vi "Perform Measurement.vi"(7 "MeasurementConfiguration":T2={"BandStart"=20.0, "BandStop"=20000.0, "Amplitude"=1.0, "Frequency"=1000.0, "FullScaleRange"=2.825, "DataLine"=0, "SampleRate"=12288000, "MeasurementDuration"=19200.0, "Channel"=0, "FrameSyncEdgeForChannel_0"=0, "ChannelCountPerFrame"=2, "ChannelLength"=32, "BitDepth"=24, "Channel_0_offset"=1, "Endianness"=0, "DataJustification"=0, "FrameSyncPulseWidth"=32, "BitClockEdgeSync"=1, "ClockRate"=0, "FrameLength"=0, "NumberOfWords"=0, "Sensitivity"=0.0}, 8 "Y":dbl[](array[numeric]), 9 "dt":dbl, 11 "WeightingFilter":string) -> (1 "error out":errorcluster, 2 "TimeDomain":dbl[](array[numeric]), 3 "Spectrum":dbl[](array[numeric]), 5 "MeasurementResults":T1)   [LabVIEW 2021]
uses:
  Measurement Configuration.ctl
  MeasurementResults.ctl
  <vilib>/addons/_NISVFA/_Shared subVIs/Controls/svc_Window.ctl
  <vilib>/addons/_NISVFA/_Shared subVIs/Common/SVL Set dB Reference (N Ch - 1 Ref).vi
  <vilib>/addons/Sound and Vibration/svt_Level/SVL AC & DC Level (Time) (N Ch).vi
  <vilib>/addons/Sound and Vibration/svt_Single Tone Measurements/SVT Spurious Free Dynamic Range (Frequency) (1 Ch).vi
  <vilib>/addons/_NISVFA/_Spectrum Processing/SVFA Unit Conversion (Complex) (1 Ch).vi
  <vilib>/addons/_NISVFA/_Shared subVIs/Common/SVL Set dB Reference (1 Ch).vi
  <vilib>/addons/Sound and Vibration/svt_Level/SVL AC & DC Level (Time) (1 Ch).vi
  <vilib>/addons/_NISVFA/_Spectrum Processing/SVFA Get Spectrum Subset.vi
  <vilib>/addons/_NISVFA/_Spectrum Processing/SVFA Get Spectrum Subset (Complex) (1 Ch).vi
  <vilib>/addons/_NISVFA/_Shared subVIs/Common/svc_Window Parameters.vi
  <vilib>/addons/_NISVFA/_Shared subVIs/Common/svc_Extract Single Tone Information (complex).vi
  <vilib>/addons/_NISVFA/_Shared subVIs/Common/svc_Check Frequency Range in Spectrum.vi
  <vilib>/addons/_NISVFA/_Spectrum Processing/SVFA Spectrum Peak Search.vi
  <vilib>/addons/_NISVFA/_Spectrum Processing/SVFA Spectrum Peak Search (1 Ch).vi
  <vilib>/addons/_NISVFA/_Shared subVIs/Common/svc_Spectrum Units.vi
  <vilib>/addons/_NISVFA/_Shared subVIs/Common/svc_Log View for Spectrum (1Ch).vi
  <vilib>/addons/_NISVFA/_Spectrum Processing/SVFA Unit Conversion (1 Ch).vi
  <vilib>/addons/_NISVFA/_Shared subVIs/Common/svc_Complex Datatype Defaults.vi
  <vilib>/addons/_NISVFA/_Shared subVIs/Common/svc_Build Unit Label for Frequency Range.vi
  <vilib>/addons/_NISVFA/_Shared subVIs/Common/SVL Set dB Reference (variant).vi
  <vilib>/addons/_NISVFA/_Shared subVIs/Common/svc_Get SV Channel Info.vi
  <vilib>/Analysis/baseanly.llb/Mean.vi
  <vilib>/Analysis/baseanly.llb/Mean (DBL).vi
  <vilib>/addons/_NISVFA/_Shared subVIs/Windowing/svfa_Scaled Time Domain Window (Array).vi
  <vilib>/addons/_NISVFA/_Spectrum Processing/SVFA Get Tone Amplitude and Phase (1 Ch).vi
  <vilib>/addons/_NISVFA/_Spectrum Processing/subVIs/svfa_Compute Complex Spectrum for Export.vi
  <vilib>/addons/_NISVFA/_Shared subVIs/Common/svc_Check Frequency Range in Bandwidth.vi
  <vilib>/addons/_NISVFA/_Shared subVIs/Common/svc_Convert Start and Stop to Start Index and Length.vi
  <vilib>/addons/_NISVFA/_Spectrum Processing/subVIs/svfa_Spectrum Peak Search.vi
  <vilib>/addons/_NISVFA/_Shared subVIs/Common/svc_Format Value (DBL).vi
  <vilib>/addons/_NISVFA/_Shared subVIs/Common/svc_Get Weighting Enum and Labels.vi
  <vilib>/addons/_NISVFA/_Shared subVIs/Common/svc_Engineering Units to Unit Label.vi
  <vilib>/addons/_NISVFA/_Shared subVIs/Common/svc_Surround NonAlpha String with Parentheses.vi
  <vilib>/dlg_ctls.llb/Space Constant.vi
  <vilib>/addons/_NISVFA/_Shared subVIs/Common/svc_Unwrap Phase.vi
  <vilib>/addons/_NISVFA/_Shared subVIs/Common/svc_Convert Spectrum Array to dB.vi
  <vilib>/addons/_NISVFA/_Spectrum Processing/subVIs/svfa_Conversion Utility (spectrum info).vi
  <vilib>/addons/_NISVFA/_Shared subVIs/Common/svc_Unit Label to Engineering Units.vi
  <vilib>/addons/_NISVFA/_Spectrum Processing/subVIs/svfa_Spectrum Info Window to windowTd Type Def.vi
  <vilib>/Analysis/4window.llb/Force Window.vi
  <vilib>/Analysis/4window.llb/Force Window (DBL).vi
  <vilib>/Analysis/4window.llb/Exponential Window.vi
  <vilib>/Analysis/4window.llb/Exponential Window (DBL).vi
  <vilib>/addons/_NISVFA/_Spectrum Processing/subVIs/svfa_Window Frequency Response.vi
  <vilib>/addons/_NISVFA/_Spectrum Processing/subVIs/svfa_Window Frequency Response (double array).vi
  <vilib>/Analysis/baseanly.llb/Dot Product.vi
  <vilib>/Analysis/baseanly.llb/Complex Dot Product.vi
  <vilib>/addons/_NISVFA/_Spectrum Processing/subVIs/svfa_Peak Rough Search Indices.vi
  <vilib>/addons/_NISVFA/_Shared subVIs/Common/svc_Unit Label Lexical Class.vi
  <vilib>/addons/_NISVFA/_Spectrum Processing/subVIs/svfa_Peak to RMS to Peak2Peak.vi
  <vilib>/addons/_NISVFA/_Spectrum Processing/subVIs/svfa_Mag to Mag2.vi
  <vilib>/addons/_NISVFA/_Spectrum Processing/subVIs/svfa_Linear to dB.vi
  <vilib>/addons/_NISVFA/_Spectrum Processing/subVIs/svfa_dBrefA to dBrefB.vi
  <vilib>/addons/_NISVFA/_Spectrum Processing/subVIs/svfa_Spectrum to Spectral Density.vi
  <vilib>/addons/_NISVFA/_Spectrum Processing/subVIs/svfa_Rect Window Frequency Response.vi
  <vilib>/addons/_NISVFA/_Spectrum Processing/subVIs/svfa_Cosine Window Coefficients.vi
  <vilib>/addons/Sound and Vibration/svt_Weighting/SVT Weighting Filter (N Ch).vi
  <vilib>/addons/_NISVFA/_Shared subVIs/Common/svc_Caller VI Returned in Error Source.vi
  <vilib>/addons/_NISVFA/_Shared subVIs/Common/svc_Get Window Info.vi
  <vilib>/Analysis/0measdsp.llb/Scaled Time Domain Window.vi
  <vilib>/Analysis/0measdsp.llb/Scaled Time Domain Window (DBL).vi
  <vilib>/Utility/error.llb/Error Cluster From Error Code.vi
  <vilib>/Analysis/baseanly.llb/Std Deviation and Variance.vi
  <vilib>/addons/Sound and Vibration/svt_Single Tone Measurements/SVT Gain (Time) (1 Ch).vi
  <vilib>/addons/Sound and Vibration/svt_Distortion/SVT SNR without Harmonics (Frequency) (1 Ch).vi
  <vilib>/addons/Sound and Vibration/svt_Single Tone Measurements/SVT Dynamic Range (Frequency) (1 Ch).vi
  <vilib>/addons/Sound and Vibration/svt_Distortion/subVIs/sv_Check Data Valid (Audio) (1 Ch).vi
  <vilib>/addons/_NISVFA/_Shared subVIs/Common/svc_Convert Frequency to Frequency String.vi
  <vilib>/Analysis/4window.llb/window parameters.vi
  <vilib>/Analysis/4window.llb/Window Properties.vi
  <vilib>/Analysis/4window.llb/Window Properties by Name.vi
  <vilib>/addons/_NISVFA/_Spectrum Processing/subVIs/svfa_Spectrum Peak Tone Search and Estimation (complex).vi
  <vilib>/measure/masignal.llb/Tones and Noise Waveform.vi
  <vilib>/addons/_NISVFA/_Shared subVIs/Common/svc_FFT with Window.vi
  <vilib>/Analysis/1siggen.llb/Square Wave.vi
  <vilib>/addons/_NISVFA/_Spectrum Processing/subVIs/svfa_Three Finger Peak Search.vi
  <vilib>/addons/Sound and Vibration/svt_Distortion/subVIs/sv_Peak View Amplitude (1 Ch).vi
  <vilib>/addons/Sound and Vibration/svt_Single Tone Measurements/SoundVib_SingleTone.lvlib
  <vilib>/addons/Sound and Vibration/svt_Distortion/SoundVib_Distortion.lvlib
  <vilib>/addons/Sound and Vibration/svt_Weighting/SoundVib_ABCWeighting.lvlib
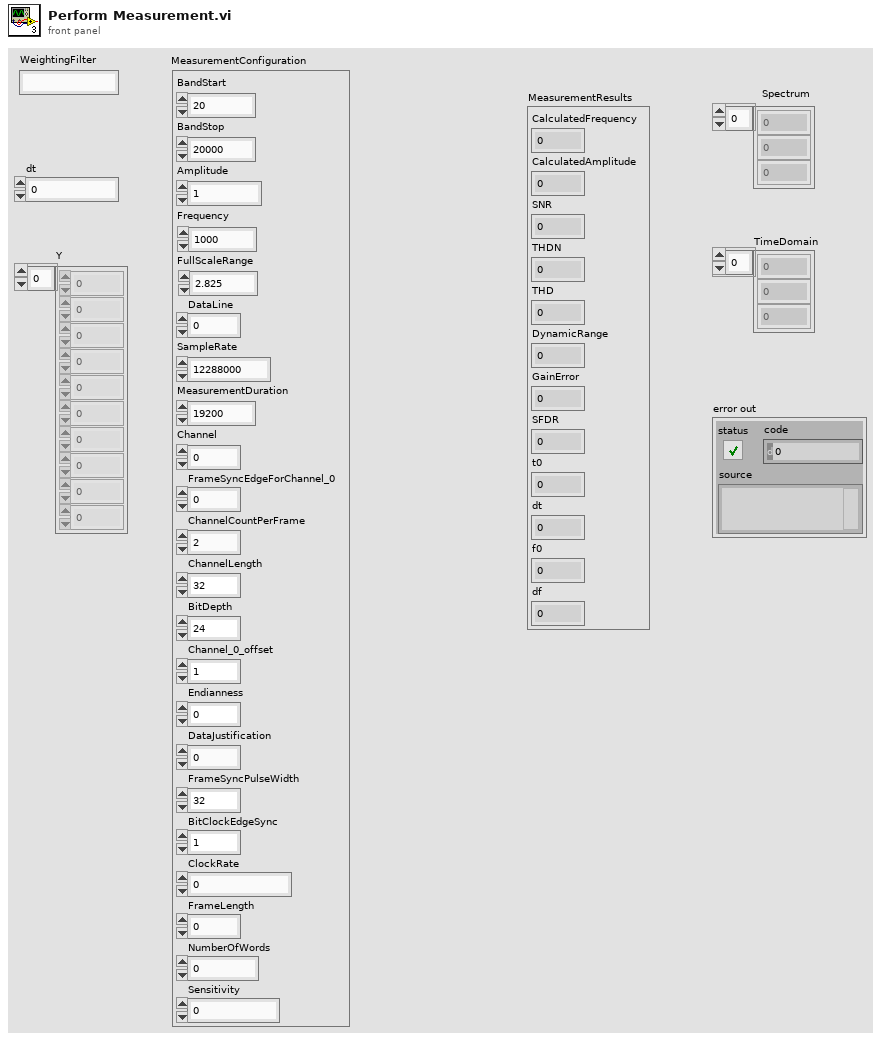
[diagram p1: front panel]
types:
  T1 = typedef "MeasurementResults.ctl" = cluster{"CalculatedFrequency":dbl, "CalculatedAmplitude":dbl, "SNR":dbl, "THDN":dbl, "THD":dbl, "DynamicRange":dbl, "GainError":dbl, "SFDR":dbl, "t0":dbl, "dt":dbl, "f0":dbl, "df":dbl}
  T2 = typedef "Measurement Configuration.ctl" = cluster{"BandStart":dbl, "BandStop":dbl, "Amplitude":dbl, "Frequency":dbl, "FullScaleRange":dbl, "DataLine":u32, "SampleRate":u32, "MeasurementDuration":dbl, "Channel":u32, "FrameSyncEdgeForChannel_0":u32, "ChannelCountPerFrame":u32, "ChannelLength":u32, "BitDepth":u32, "Channel_0_offset":u32, "Endianness":u32, "DataJustification":u32, "FrameSyncPulseWidth":u32, "BitClockEdgeSync":u32, "ClockRate":u32, "FrameLength":u32, "NumberOfWords":u32, "Sensitivity":dbl}
  T3 = cluster{"start frequency":dbl, "stop frequency":dbl}
  T4 = enum16{"no change", "spectrum", "spectral density"}
  T5 = cluster{"linear/dB":enum16{"no change", "linear", "dB"}, "dB reference (0: no change)":dbl, "power/magnitude":enum16{"no change", "power", "magnitude"}, "view":enum16{"no change", "rms", "peak", "peak-peak"}}
  T6 = cluster{"gain units":enum16{"dB", "linear ratio"}, "detected fundamental amplitude units":enum16{"EU rms", "EU peak", "EU peak-peak"}}
  T7 = typedef "svc_Window.ctl" = u32
  T8 = cluster{"SNR units":enum16{"dB", "linear ratio", "%"}, "detected fundamental amplitude units":enum16{"EU rms", "EU peak", "EU peak-peak"}}
  T9 = typedef "svc_Spectrum Info.ctl" = cluster{"channel name":string, "description":string, "x-axis units":T10, "spectral info":cluster{"spectrum type":T11, "linear/dB":enum16{"linear", "dB"}, "window":u16, "window size":i32, "FFT size":i32}, "engineering units":T12, "custom label":string, "dB reference [EU]":dbl, "peak units":enum16{"rms", "peak", "peak-peak"}, "weighting filter":T13, "spectral density?":bool, "unit label":string, "spectrum skewed?":bool, "complimentary spectrum units":T14}
  T10 = typedef "svc_X-Axis Units.ctl" = u16
  T11 = typedef "svc_Spectrum Type.ctl" = enum16{"FFT Spectrum [complex]", "Amplitude [Magnitude]", "Power [Magnitude^2]", "Cross Spectrum [complex]", "Frequency Response [Complex]"}
  T12 = typedef "svc_Engineering Units Text Ring.ctl" = u16
  T13 = typedef "svc_Weighting Filter Text Ring.ctl" = u16
  T14 = typedef "svc_Complimentary Spectrum Units.ctl" = enum16{"none", "radians", "degrees", "cycles", "imaginary"}
  T15 = cluster{"complex spectrum response":cluster{"f0":dbl, "df":dbl, "complex spectrum":cdb[]}, "spectrum info":T9}
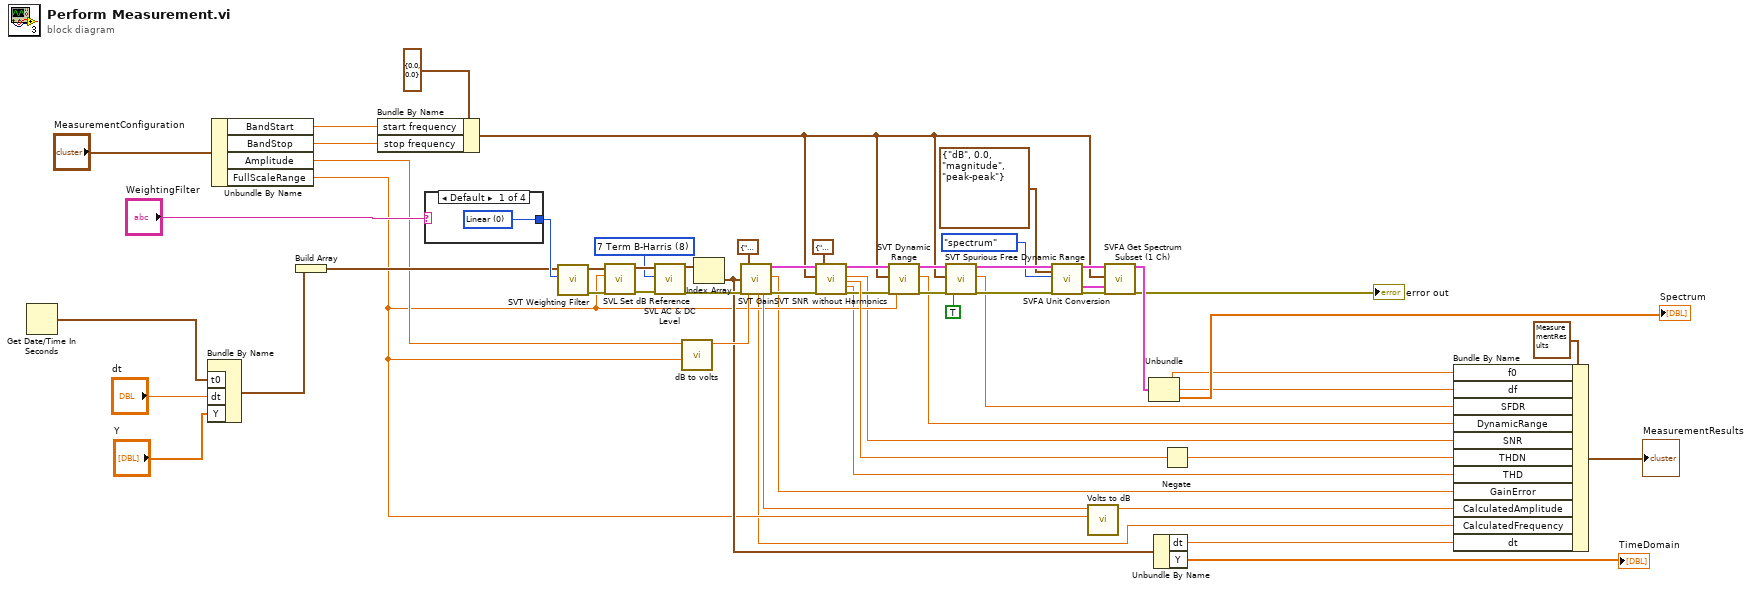
[diagram p0: block diagram]
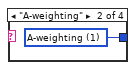
[diagram p2: hidden frame]
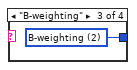
[diagram p3: hidden frame]
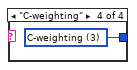
[diagram p4: hidden frame]
diagram:
  w43 = T7 8 items=["None"=0, "Hanning"=1, "Hamming"=2, "Blackman-Harris"=3, "Exact Blackman"=4, "Blackman"=5, "Flat Top"=6, "4 Term B-Harris "=7, "7 Term B-Harris"=8, "Low Sidelobe"=9, "Force"=64, "Exponential"=65, "Blackman Nuttall"=11, "Triangle"=30, "Bartlett-Hanning"=31, "Bohman"=32, "Parzen"=33, "Welch"=34, "Kaiser"=60, "Dolph-Chebyshev"=61, "Gaussian"=62] ("window")
  n1 = Get Date/Time In Seconds() -> (seconds since 1Jan1904=w1:timestamp)
  n2 = Bundle By Name ("Build Waveform")("t0"=w1, "dt"="dt", "Y"="Y") -> (w22:waveform(dbl))  [unwired: 1 in]
  n3 = Unbundle By Name("MeasurementConfiguration") -> ("BandStart"=w18:dbl, "BandStop"=w17:dbl, "Amplitude"=w16:dbl, "FullScaleRange"=w15:dbl)
  n4 = Build Array(w22) -> (w21:waveform(dbl)[])
  n5 = Bundle By Name(cluster=T3 {"start frequency"=0.0, "stop frequency"=0.0} ("frequency range"), "start frequency"=w18, "stop frequency"=w17) -> (w32:T3)
  n6 = case shown="Default" "WeightingFilter" {
    tunnel: [w59 w60 w61 w62] -> w27
    frame Default {
      w59 = u16 0 items=["Linear", "A-weighting", "B-weighting", "C-weighting"] ("weighting")
    }
    frame "A-weighting" {
      w60 = u16 1 items=["Linear", "A-weighting", "B-weighting", "C-weighting"] ("weighting")
    }
    frame "B-weighting" {
      w61 = u16 2 items=["Linear", "A-weighting", "B-weighting", "C-weighting"] ("weighting")
    }
    frame "C-weighting" {
      w62 = u16 3 items=["Linear", "A-weighting", "B-weighting", "C-weighting"] ("weighting")
    }
  }
  n7 = call-poly <vilib>:"SVT Weighting Filter.vi"("weighting"=w27, "scaled signals [EU]"=w21) -> ("error out"=w57:errorcluster, "weighted signals [EU]"=w56:waveform(dbl)[])  [unwired: 7 in]
  n8 = call-poly <vilib>:"SVL Set dB Reference.vi"("error in (no error)"=w57, "dB reference [EU]"=w15, "scaled signals in [EU]"=w56) -> ("error out"=w44:errorcluster, "scaled signals out [EU]"=w46:waveform(dbl)[])  [unwired: 7 in]
  n9 = call-poly <vilib>:"SVL AC & DC Level.vi"("scaled signals in [EU]"=w46, "window"=w43, "error in (no error)"=w44) -> ("AC signals [EU]"=w45:waveform(dbl)[], "error out"=w52:errorcluster)  [unwired: 11 in, 4 out]
  n10 = call "dB to volts.vi"("Full scale range"=w15, "Voltage(dB)"=w16) -> ("Voltage(volts)"=w35:dbl)  [unwired: 9 in]
  n11 = Index Array(array=w45) -> (element=w26:waveform(dbl))  [unwired: 1 in]
  n12 = call-poly <vilib>:"SVT Gain.vi"("scaled signal [EU]"=w26, "error in (no error)"=w52, "desired units"=T6 {"gain units"=enum."dB", "detected fundamental amplitude units"=enum."EU peak"}, "amplitude [EU peak]"=w35) -> ("detected fundamental\nfrequency [Hz]"=w3:dbl, "detected fundamental\namplitude"=w34:dbl, "complex spectrum"=w41:T15, "gain"=w5:dbl, "error out"=w42:errorcluster)  [unwired: 10 in, 1 out]
  n13 = call-poly <vilib>:"SVT SNR without Harmonics.vi"("complex spectrum"=w41, "frequency range"=w32, "error in (no error)"=w42, "desired units"=T8 {"SNR units"=enum."dB", "detected fundamental amplitude units"=enum."EU rms"}) -> ("complex spectrum"=w48:T15, "SNR (without harmonics)"=w8:dbl, "SINAD"=w49:dbl, "THD"=w6:dbl, "error out"=w47:errorcluster)  [unwired: 8 in, 3 out]
  n14 = call-poly <vilib>:"SVT Dynamic Range.vi"("complex spectrum"=w48, "frequency range"=w32, "error in (no error)"=w47, "full scale amplitude [EU peak]"=w15) -> ("dup complex spectrum"=w53:T15, "dynamic range"=w9:dbl, "error out"=w54:errorcluster)  [unwired: 10 in, 3 out]
  n15 = call-poly <vilib>:"SVT Spurious Free Dynamic Range.vi"("complex spectrum"=w53, "frequency range"=w32, "error in (no error)"=w54, "exclude harmonics"=TRUE) -> ("complex spectrum"=w39:T15, "spurious free dynamic range"=w10:dbl, "error out"=w40:errorcluster)  [unwired: 8 in, 5 out]
  n16 = call-poly <vilib>:"SVFA Unit Conversion.vi"("complex spectrum"=w39, "desired scaling"=T5 {"linear/dB"=enum."dB", "dB reference (0: no change)"=0.0, "power/magnitude"=enum."magnitude", "view"=enum."peak-peak"}, "spectral density desired"=T4."spectrum", "error in (no error)"=w40) -> ("converted spectrum"=w33:cluster{"x0":dbl, "dx":dbl, "magnitude":dbl[]}, "spectrum info out"=w29:T9, "error out"=w28:errorcluster)  [unwired: 10 in, 3 out]
  n17 = call "Volts to dB.vi"("Full scale range"=w15, "Voltage(V)"=w34) -> ("Voltage(dB)"=w4:dbl)  [unwired: 9 in]
  n18 = call <vilib>:"SVFA Get Spectrum Subset (1 Ch).vi"("spectrum"=w33, "range"=w32, "spectrum info"=w29, "error in (no error)"=w28) -> ("spectrum subset"=w31:cluster{"x0":dbl, "dx":dbl, "magnitude":dbl[]}, "error out"=→"error out":errorcluster)  [unwired: 10 in, 4 out]
  n19 = Unbundle(w31) -> ("x0"=w12:dbl, "dx"=w11:dbl, "magnitude"=→"Spectrum":dbl[])
  n20 = Unbundle By Name ("Get Waveform Components")(w26) -> ("dt"=w2:dbl, "Y"=→"TimeDomain":dbl[])
  n21 = Negate(x=w49) -> (-x=w7:dbl)
  n22 = Bundle By Name(cluster=T1 {"CalculatedFrequency"=0.0, "CalculatedAmplitude"=0.0, "SNR"=0.0, "THDN"=0.0, "THD"=0.0, "DynamicRange"=0.0, "GainError"=0.0, "SFDR"=0.0, "t0"=0.0, "dt"=0.0, "f0"=0.0, "df"=0.0} ("Measurement Results"), "f0"=w12, "df"=w11, "SFDR"=w10, "DynamicRange"=w9, "SNR"=w8, "THDN"=w7, "THD"=w6, "GainError"=w5, "CalculatedAmplitude"=w4, "CalculatedFrequency"=w3, "dt"=w2) -> (→"MeasurementResults":T1)
